vi "About.vi"() -> ()   [LabVIEW 2013]
uses:
  <vilib>/Utility/inputDevices.llb/mouseAcquire.vi
  <vilib>/Platform/browser.llb/Open URL in Default Browser (string).vi
panel:
  in  "?":bool
  in  "Website":bool
  in  "Close":bool
  in  "ReportBug":bool
  out "Version Info.":string
  # "3d Temperature Mapping"
  # "Copyright 2015"
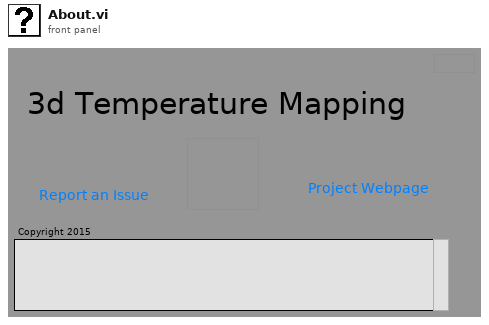
[diagram p1: front panel]
types:
  T1 = typedef "LVRectTypeDef.ctl" = cluster{"Left":i16, "Top":i16, "Right":i16, "Bottom":i16}
  T2 = cluster{"Horizontal":i32, "Vertical":i32, "Scrolling":i32}
  T3 = cluster{"button 1":bool, "button 2":bool, "button 3":bool, "button 4":bool}
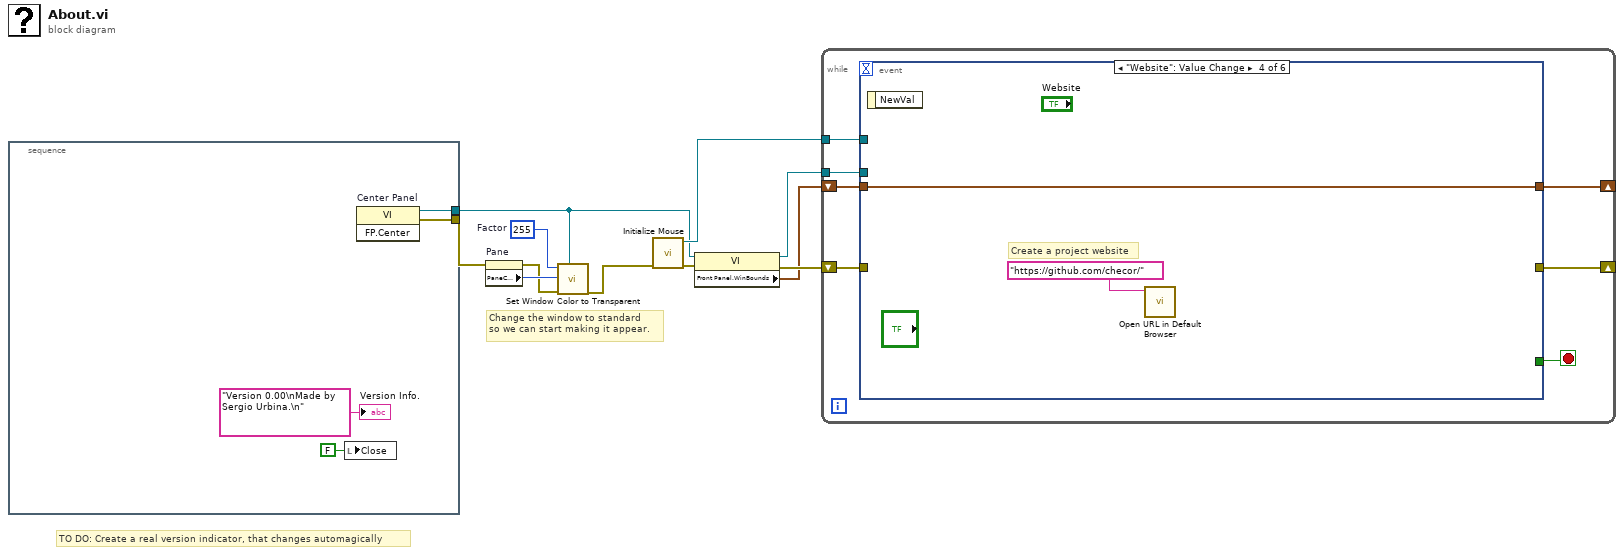
[diagram p0: block diagram]
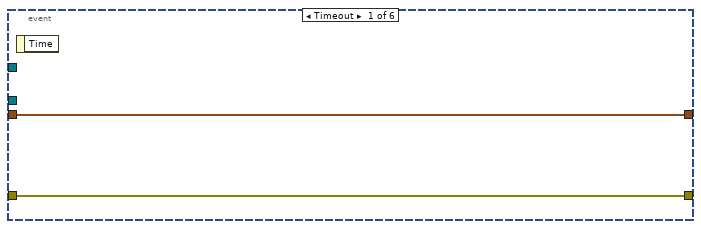
[diagram p2: hidden frame]
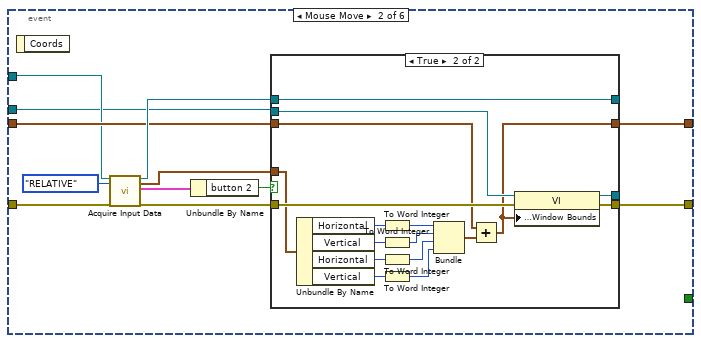
[diagram p3: hidden frame]
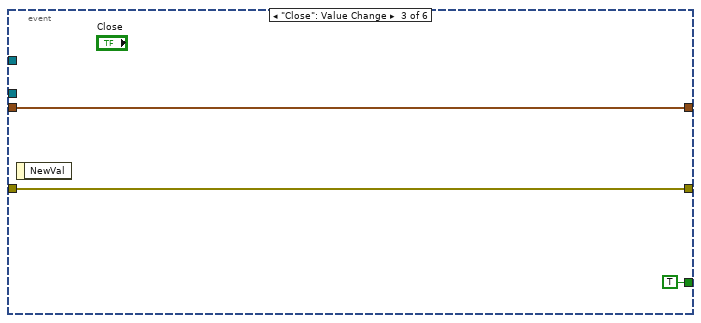
[diagram p5: hidden frame]
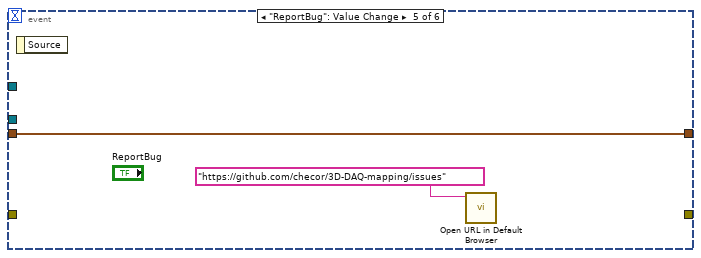
[diagram p6: hidden frame]
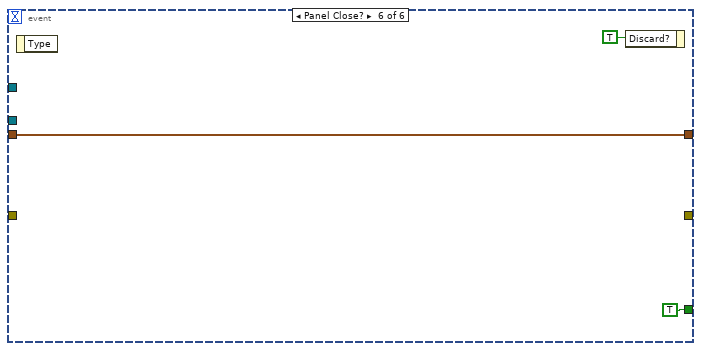
[diagram p7: hidden frame]
diagram:
  w11 = u8 255  # Factor
  # "TO DO: Create a real version indicator, that changes automagically"
  # "Change the window to standard\nso we can start making it appear."
  n1 = stacked-sequence {
    tunnel: [w14] -> w2
    tunnel: [w13] -> w1
    frame #0 {
      n2 = local write "Close"(FALSE ("Close")) -> ()
      n3 = invoke on="Center Panel" class="VI" method="FP.Center"() -> (reference out=w13:refnum<vi>, error out=w14:errorcluster)  [unwired: 3 in, 1 out]
      "Version Info." <- "Version 0.00\nMade by Sergio Urbina.\n" ("Version Info.")
    }
  }
  n4 = property on="Pane" class="Pane"(error in=w2) -> (error out=w9:errorcluster, "PaneColor"=w10:u32)  [unwired: 1 in, 1 out]
  n5 = call "Set Window Color to Transparent.vi"("Calling VI's reference"=w1, "error in (no error)"=w9, "Color to Replace"=w10, "Factor"=w11) -> ("error out"=w3:errorcluster)  [unwired: 4 in]
  n6 = call <vilib>:"Initialize Mouse.vi"("error in (no error)"=w3) -> ("error out"=w7:errorcluster, "device ID"=w8:refnum<k1>)  [unwired: 9 out]
  n7 = property class="VI"(reference=w1, error in=w7) -> (reference out=w4:refnum<vi>, error out=w6:errorcluster, "Front Panel.WinBounds"=w5:T1)
  n8 = while {
    shift-right: [w22] -> _
    shift-left: w6 -> [w17]
    tunnel: w8 -> [w19]
    tunnel: w4 -> [w18]
    shift-right: [w16] -> _
    shift-left: w5 -> [w20]
    stop <- w21 stop-if-true
    n9 = event shown="[3] \"Website\": Value Change" {
      selector: _ -> [_ _ _ _ _ _]
      dyn-events: _ -> [_ _ _ _ _ _]
      timeout: _ -> [_ _ _ _ _ _]
      tunnel: w17 -> [w24 w28 w59 _ _ _]
      tunnel: [w24 w27 w59 _ _ _] -> w22
      tunnel: [_ _ TRUE ("Close") _ _ TRUE ("Close")] -> w21
      tunnel: w20 -> [w23 w30 w58 w61 w64 w65]
      tunnel: w19 -> [_ w29 _ _ _ _]
      tunnel: w18 -> [_ w26 _ _ _ _]
      tunnel: [w23 w25 w58 w61 w64 w65] -> w16
      event Timeout {
        n10 = event-data() -> ()  [unwired: 1 in, 1 out]
      }
      event Mouse Move {
        n11 = event-data() -> ()  [unwired: 1 in, 1 out]
        n12 = call-poly <vilib>:"Acquire Input Data.vi"("device ID"=w29, "key mode"=enum16{"RELATIVE", "ABSOLUTE"}."RELATIVE", "error in (no error)"=w28) -> ("device ID"=w34:refnum<k1>, "axis info"=w36:T2, "button info"=w32:T3, "error out"=w35:errorcluster)  [unwired: 13 out]
        n13 = Unbundle By Name(w32) -> ("button 2"=w33:bool)
        n14 = case shown="True" w33 {
          tunnel: w34 -> [w40 w57]
          tunnel: w35 -> [w39 w54]
          tunnel: [w39 w55] -> w27
          tunnel: [w40 w57] -> _
          tunnel: w30 -> [w38 w43]
          tunnel: [w38 w41] -> w25
          tunnel: [w37 w56] -> _
          tunnel: w26 -> [w37 w53]
          tunnel: w36 -> [_ w52]
          frame False {
          }
          frame True {
            n15 = Unbundle By Name(w52) -> ("Horizontal"=w51:i32, "Vertical"=w50:i32, "Horizontal"=w47:i32, "Vertical"=w46:i32)
            n16 = To Word Integer(number=w51) -> (16bit integer=w49:i16)
            n17 = To Word Integer(number=w50) -> (16bit integer=w48:i16)
            n18 = To Word Integer(number=w47) -> (16bit integer=w45:i16)
            n19 = To Word Integer(number=w46) -> (16bit integer=w44:i16)
            n20 = Bundle(w49, w48, w45, w44) -> (w42:cluster{i16, i16, i16, i16})  [unwired: 1 out]
            n21 = Add(x=w43, y=w42) -> (x+y=w41:T1)
            n22 = property class="VI"(reference=w53, error in=w54, "Front Panel Window:Window Bounds"=w41) -> (reference out=w56:refnum<vi>, error out=w55:errorcluster)
          }
        }
      }
      event "Close": Value Change {
        n23 = event-data() -> ()  [unwired: 1 in, 1 out]
      }
      event "Website": Value Change {
        # "Create a project website"
        n24 = event-data() -> ()  [unwired: 1 in, 1 out]
        n25 = call-poly <vilib>:"Open URL in Default Browser.vi"("URL"="https://github.com/checor/" ("Link")) -> ()  [unwired: 5 in, 2 out]
      }
      event "ReportBug": Value Change {
        n26 = event-data() -> ()  [unwired: 1 in, 1 out]
        n27 = call-poly <vilib>:"Open URL in Default Browser.vi"("URL"="https://github.com/checor/3D-DAQ-mapping/issues" ("Link")) -> ()  [unwired: 5 in, 2 out]
      }
      event Panel Close? {
        n28 = event-data() -> ()  [unwired: 1 in, 1 out]
        n29 = event-data("Discard?"=TRUE) -> ()  [unwired: 1 in, 1 out]
      }
    }
  }
